vi "Spartan Builder - Embed Configure Restart Stub.vi"(8 "error in":errorcluster) -> (0 "error out":errorcluster)   [LabVIEW 2011]
doc: "Use this VI Template to create a custom Pre-/Post-Build VI."
uses:
  OpenG.LIB/file/file.llb/Strip Path Extension - String__ogtk.vi
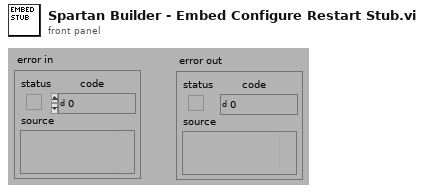
[diagram p1: front panel]
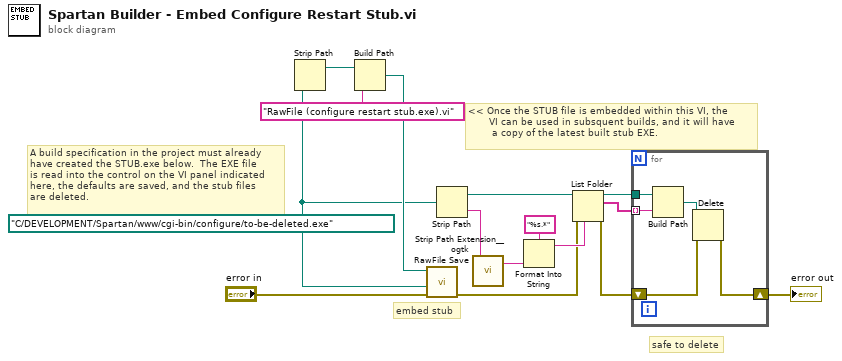
[diagram p0: block diagram]
diagram:
  w1 = path "C:/DEVELOPMENT/Spartan/www/cgi-bin/configure/to-be-deleted.exe" ("appended path")
  # "<< Once the STUB file is embedded within this VI, the\n       VI can be used in subsquent builds, and it will have\n        a copy of the latest built stub EXE."
  # "A build specification in the project must already\nhave created the STUB.exe below.  The EXE file\nis read into the control on the VI panel indicated\nhere, the defaults are saved, and the stub files\nare deleted."
  # "safe to delete"
  # "embed stub"
  n1 = Strip Path(path=w1) -> (stripped path=w14:path)  [unwired: 1 out]
  n2 = Build Path(base path=w14, name or relative path="RawFile (configure restart stub.exe).vi" ("Control Name (\"\")")) -> (appended path=w12:path)
  n3 = call "RawFile Save.vi"("error in (no error)"="error in", "File Path (empty)"=w1, "VI Path (empty)"=w12) -> ("error out"=w6:errorcluster)  [unwired: 8 out]
  n4 = Strip Path(path=w1) -> (stripped path=w11:path, name=w10:string)
  n5 = call-poly "Strip Path Extension__ogtk.vi"("path"=w10) -> ("root"=w8:string)  [unwired: 1 out]
  n6 = Format Into String(format string="%s.*" ("pattern"), w8) -> (resulting string=w7:string)  [unwired: 2 in, 1 out]
  n7 = List Folder(path=w11, pattern=w7, error in=w6) -> (path out=w5:path, filenames=w4:string[], error out=w3:errorcluster)  [unwired: 2 out]
  n8 = for {
    tunnel: w5 -> [w20]
    tunnel: w4 -> [w19] mode=indexing
    shift-right: [w16] -> w2
    shift-left: w3 -> [w17]
    n9 = Build Path(base path=w20, name or relative path=w19) -> (appended path=w18:path)
    n10 = Delete(path (use dialog)=w18, error in=w17) -> (error out=w16:errorcluster)  [unwired: 5 out]
  }
  "error out" <- w2
